vi "Driver Update Table.vi"(4 "error in (no error)":errorcluster, 6 "New Test Record":T2, 7 "Connection Refnum":T1) -> (0 "error out":errorcluster, 3 "Connection Refnum":T1)   [LabVIEW 2011]
uses:
  Driver Record.ctl
  SI.LIB/ODBC/SQL Controls/Connection Refnum.ctl
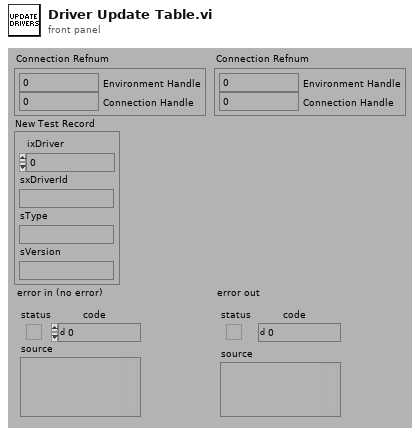
[diagram p1: front panel]
types:
  T1 = typedef "Connection Refnum.ctl" = cluster{"Environment Handle":i32, "Connection Handle":i32}
  T2 = typedef "Driver Record.ctl" = cluster{"ixDriver":i32, "sxDriverId":string, "sType":string, "sVersion":string}
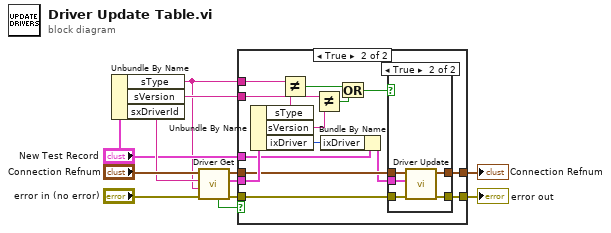
[diagram p0: block diagram]
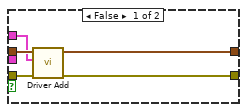
[diagram p2: hidden frame]
diagram:
  n1 = Unbundle By Name("New Test Record") -> ("sType"=w4:string, "sVersion"=w10:string, "sxDriverId"=w9:string)
  n2 = call "Driver Get.vi"("error in (no error)"="error in (no error)", "sType"=w4, "sxDriverId"=w9, "Connection Refnum"="Connection Refnum") -> ("error out"=w6:errorcluster, "Driver Record"=w11:T2, "Connection Refnum"=w8:T1, "Data Present"=w5:bool)  [unwired: 4 out]
  n3 = case shown="True" w5 {
    tunnel: w11 -> [_ w32]
    tunnel: w4 -> [_ w31]
    tunnel: w10 -> [_ w29]
    tunnel: w8 -> [w17 w25]
    tunnel: "New Test Record" -> [w13 w24]
    tunnel: w6 -> [w16 w21]
    tunnel: [w14 w20] -> w1
    tunnel: [w15 w19] -> w2
    frame False {
      n4 = call "Driver Add.vi"("error in (no error)"=w16, "Driver Record"=w13, "Connection Refnum"=w17) -> ("error out"=w15:errorcluster, "Connection Refnum"=w14:T1)  [unwired: 7 out]
    }
    frame True {
      n5 = Unbundle By Name(w32) -> ("sType"=w30:string, "sVersion"=w28:string, "ixDriver"=w23:i32)
      n6 = Not Equal?(x=w31, y=w30) -> (x != y?=w27:bool)
      n7 = Not Equal?(x=w29, y=w28) -> (x != y?=w26:bool)
      n8 = Bundle By Name(cluster=w24, "ixDriver"=w23) -> (w22:T2)
      n9 = Or(x=w27, y=w26) -> (x .or. y?=w18:bool)
      n10 = case shown="True" w18 {
        tunnel: w25 -> [w34 w39]
        tunnel: w22 -> [_ w38]
        tunnel: w21 -> [w33 w37]
        tunnel: [w34 w36] -> w20
        tunnel: [w33 w35] -> w19
        frame False {
        }
        frame True {
          n11 = call "Driver Update.vi"("error in (no error)"=w37, "Driver Record"=w38, "Connection Refnum"=w39) -> ("error out"=w35:errorcluster, "Connection Refnum"=w36:T1)  [unwired: 7 out]
        }
      }
    }
  }
  "error out" <- w2
  "Connection Refnum" <- w1
